vi "Config From JSON.vi"(7 "Mutable (F)":bool, 8 "error in (no error)":errorcluster, 10 "JSON":string) -> (0 "error out":errorcluster, 2 "Config":refnum<class "Config Manager.lvclass">)   [LabVIEW 2023, in "CDM-Config.lvlib" / "Config-JSON.lvclass"]
uses:
  Config-JSON.lvclass
  Config Manager/Config Manager.lvclass
  Config-JSON.lvclass/Config-JSON.ctl
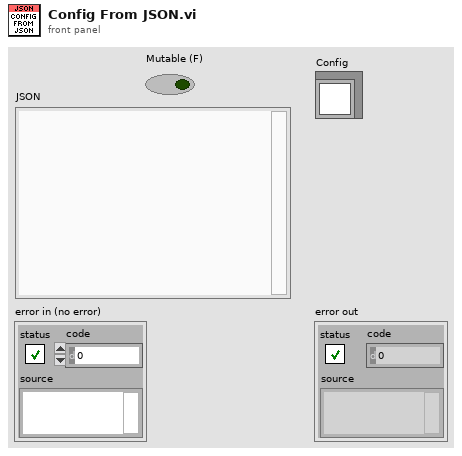
[diagram p1: front panel]
types:
  T1 = typedef "CDM-Config.lvlib/Config Element.ctl" = cluster{"Hierarchy":string[], "Value":variant, "Meta Data":T2[], "Value Type":T3, "Child Order":i32}
  T2 = typedef "CDM-Config.lvlib/Meta Data.ctl" = cluster{"Name":string, "Value":string}
  T3 = typedef "CDM-Config.lvlib/Value Type.ctl" = enum16{"String", "Number", "Bool", "Object", "Array"}
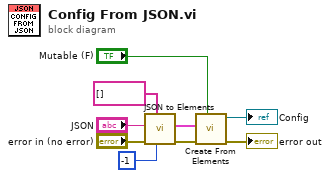
[diagram p0: block diagram]
diagram:
  n1 = call "JSON to Elements.vi"("Child Order"=-1, "Hierarchy"=string[] [] ("Parent Hierarchy"), "error in (no error)"="error in (no error)", "JSON"="JSON") -> ("error out"=w6:errorcluster, "Elements"=w5:T1[])  [unwired: 6 in]
  n2 = call "Create From Elements.vi"("Mutable (F)"="Mutable (F)", "error in (no error)"=w6, "Elements"=w5) -> ("error out"=→"error out":errorcluster, "Config Manager out"=→"Config":refnum<class "Config Manager.lvclass">)  [unwired: 7 in]
